vi "DataFinder_DisplaySignal_nointerps.vi"(8 "error in":errorcluster {"code" min=0 max=0}, 10 "result references":refnum<k20>[](array[refnum])) -> ()   [LabVIEW 2014]
doc: "Displays resulting signals as waveforms."
uses:
  <vilib>/DataFinder/DataTypes/property.ctl
  <vilib>/DataFinder/DataTypes/object type.ctl
  <vilib>/DataFinder/DataTypes/data type.ctl
  <vilib>/DataFinder/Get Property Values (Numeric Property).vi
  <vilib>/DataFinder/Get Property Values (Date Property).vi
  <vilib>/Utility/error.llb/DialogType.ctl
  <vilib>/DataFinder/NI_DataFinder Toolkit.lvlib
  <vilib>/DataFinder/Results to Waveforms (ddt).vi
  <vilib>/Analysis/NI_AALPro.lvlib
panel:
  out "Array":i32[](array[numeric])
  out "slope":dbl
  out "XY Graph 2":T1(graph)
  out "date/time string":string
  out "error out":errorcluster
  out "Timestamp":timestamp[](array[timestamp])
  out "property values":dbl[](array[numeric])
  out "XY Graph":T2(graph)
  out "Resulting Signals":dynamicdata(graph)
  out "error text":string=" INSTRUCTIONS:\r\rNormal Use:  When using subVIs that incorporate the error in/error out (or error I/O) structure, place this handler where you want to inform the user of an error, typically at the end of the I/O data path, as the last action of the program.  If the error in error? is ERROR, the handler creates a message describing the error and its source.  If the type of dialog = 1 (default), the message is displayed to the user, who can only acknowedge it.  If the type = 2, the user can acknowledge the message or abort execution; aborting a program with active I/O is not recommended.  If the type = 0, no message is displayed; this is used to process the error programmatically, and the error out cluster elements are wired to individual terminals for that reason.  \r\rOther Use:\n\r\nlocal testing.  To test the error code of a subVI or function that does not have the error I/O structure, you can wire its error code and a source string to the local error code and error source inputs.  If error in error? indicates no error and error code is not equal to 0, the local code and source are substituted for the error in values, and error? is set TRUE (ERROR)."
  in  "Close":bool
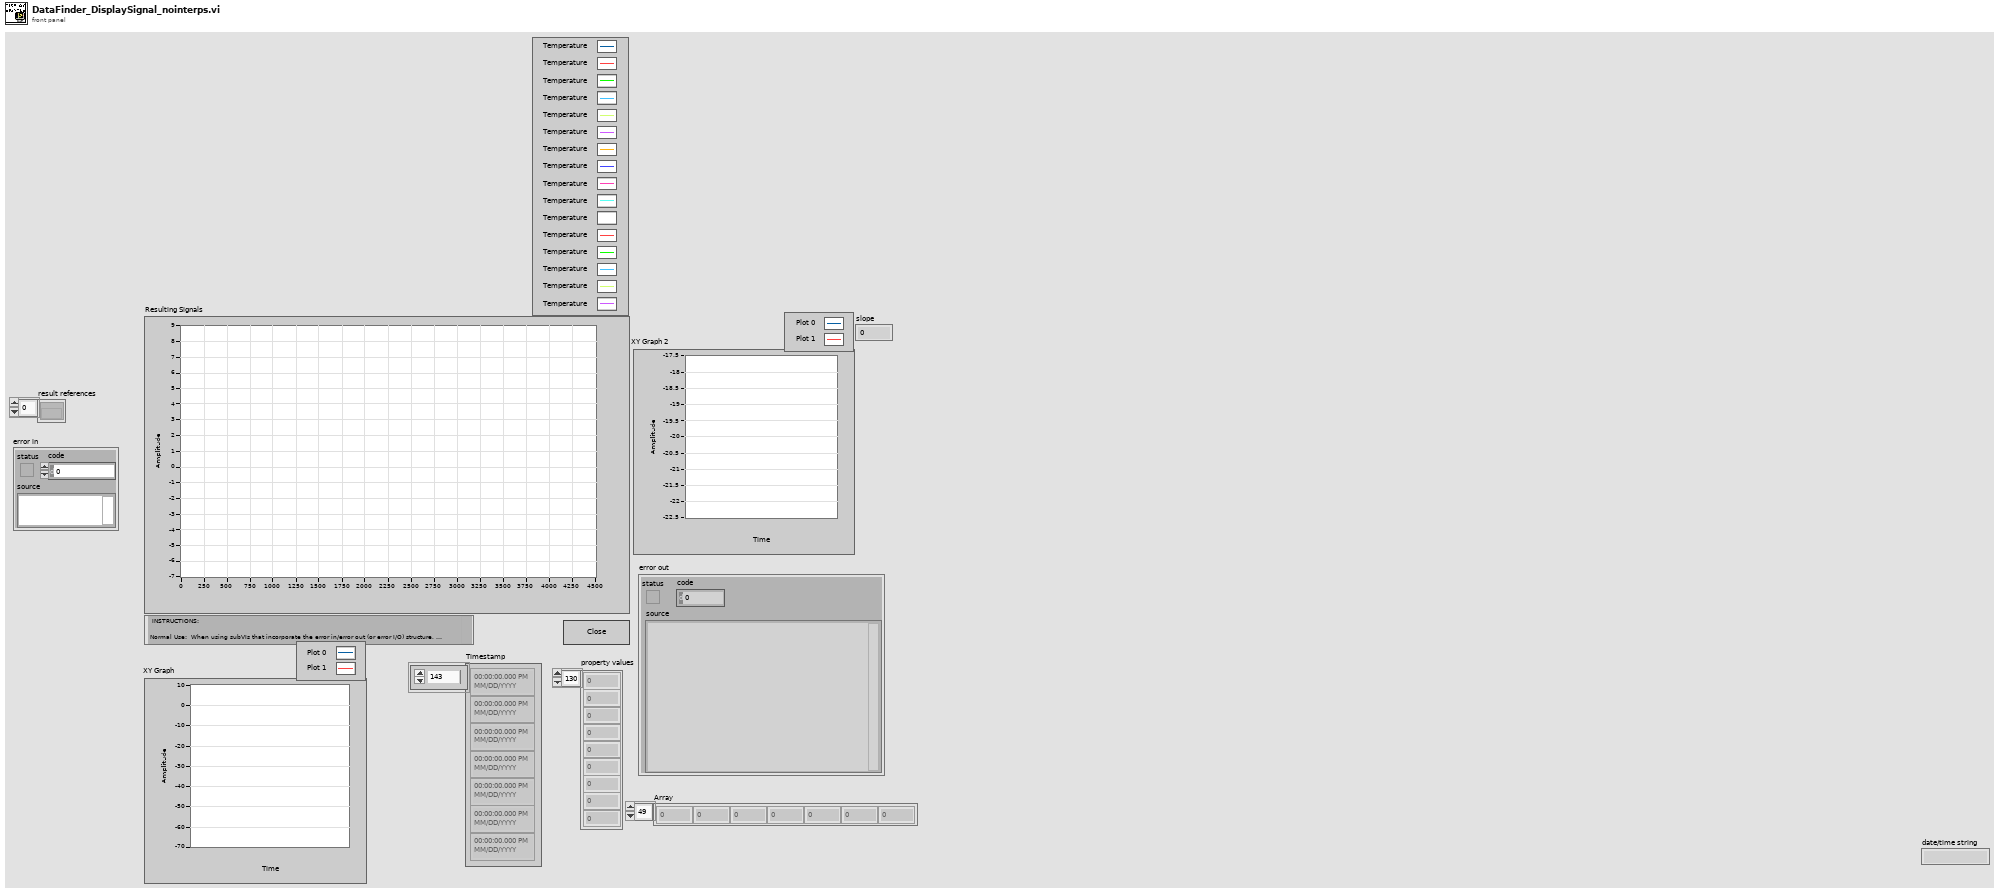
[diagram p1: front panel]
types:
  T1 = cluster{"property values":timestamp[], "Best Linear Fit":dbl[]}
  T2 = cluster{"property values":timestamp[], "Best Linear Fit":dbl[]}[]
  T3 = typedef "NI_DataFinder Toolkit.lvlib/property.ctl" = cluster{"object type":T4, "property name":string, "data type":T5}
  T4 = typedef "NI_DataFinder Toolkit.lvlib/object type.ctl" = u16
  T5 = typedef "NI_DataFinder Toolkit.lvlib/data type.ctl" = u16
  T6 = typedef "DialogType.ctl" = u16
  T7 = typedef "NI_DataFinder Controls.lvlib/DFSearchResult.ctl" = refnum<k20>
  T8 = cluster{"property values":timestamp[], "property values":dbl[]}
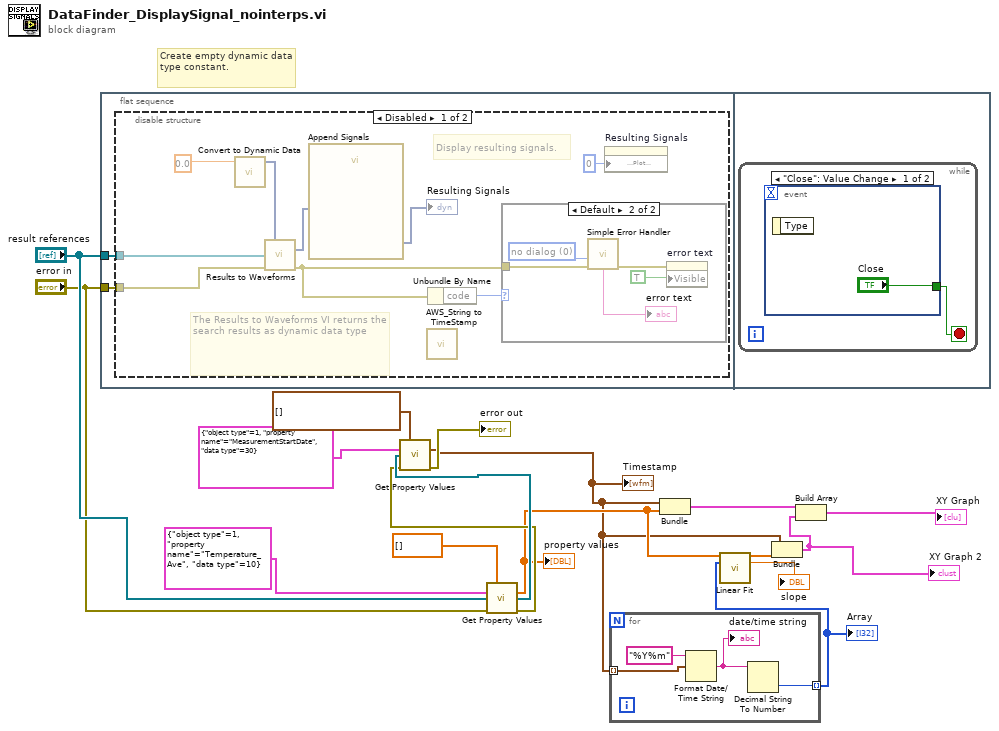
[diagram p0: block diagram]
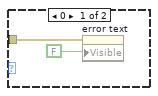
[diagram p2: hidden frame]
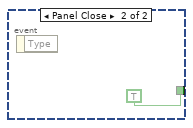
[diagram p4: hidden frame]
diagram:
  # "Create empty dynamic data type constant."
  n1 = flat-sequence {
    tunnel: "result references" -> [w19]
    tunnel: "error in" -> [w18]
    frame #0 {
      n2 = disable-structure shown="Disabled" {
        disable-tunnel: w19 -> [w26 _]
        disable-tunnel: w18 -> [w25 _]
        frame Disabled {
          # "The Results to Waveforms VI returns the search results as dynamic data type"
          # "Display resulting signals."
          n3 = call "Convert to Dynamic Data"("Double"=0.0) -> ("Dynamic Data Type"=w23:dynamicdata)  [unwired: 3 in]
          n4 = call-poly <vilib>:"Results to Waveforms.vi"("data type"=w23, "result references"=w26, "error in (no error)"=w25) -> ("signals out"=w22:dynamicdata, "error out"=w28:errorcluster)  [unwired: 11 out]
          n5 = call "Append Signals"("Input Signal A"=w22) -> ("Appended Signals"=→"Resulting Signals":dynamicdata)  [unwired: 9 in, 1 out]
          n6 = call "AWS_String to TimeStamp.vi"() -> ()  [unwired: 10 in, 1 out]
          n7 = Unbundle By Name(w28) -> ("code"=w27:i32)
          n8 = case shown="Default" w27 {
            tunnel: w28 -> [w29 w31]
            frame 0 {
              n9 = property on="error text" class="Str"(error in=w29, "Visible"=FALSE) -> ()  [unwired: 1 in, 2 out]
            }
            frame Default {
              w35 = T6 0 items=["no dialog", "OK message", "continue or stop message", "OK message + warnings", "continue/stop + warnings"] ("type of dialog (OK msg:1)")
              n10 = call <vilib>:"Simple Error Handler.vi"("type of dialog (OK msg:1)"=w35, "error in (no error)"=w31) -> ("error out"=w32:errorcluster, "message"=→"error text":string)  [unwired: 2 in, 4 out]
              n11 = property on="error text" class="Str"(error in=w32, "Visible"=TRUE) -> ()  [unwired: 1 in, 2 out]
            }
          }
          n12 = property on="Resulting Signals" class="WFGraph (strict)"("Plot.Plot Interpolation"=u8 0) -> ()  [unwired: 2 in, 2 out]
        }
        frame Enabled {
        }
      }
    }
    frame #1 {
      n13 = while {
        stop <- w36 stop-if-true
        n14 = event shown="[0] \"Close\": Value Change" {
          selector: _ -> [_ _]
          dyn-events: _ -> [_ _]
          timeout: _ -> [_ _]
          tunnel: ["Close" TRUE ("Cancel")] -> w36
          event "Close": Value Change {
            n15 = event-data() -> ()  [unwired: 1 in, 1 out]
          }
          event Panel Close {
            n16 = event-data() -> ()  [unwired: 1 in, 1 out]
          }
        }
      }
    }
  }
  n17 = call-poly <vilib>:"Get Property Values.vi"("data type"=dbl[] [], "property"=T3 {"object type"=1, "property name"="Temperature_Ave", "data type"=10}, "result references"="result references", "error in (no error)"="error in") -> ("property values"=w8:dbl[], "result references out"=w11:T7[], "error out"=w10:errorcluster)  [unwired: 9 in]
  "property values" <- w8
  n18 = call-poly <vilib>:"Get Property Values.vi"("data type"=timestamp[] [] ("Timestamp"), "property"=T3 {"object type"=1, "property name"="MeasurementStartDate", "data type"=30}, "result references"=w11, "error in (no error)"=w10) -> ("property values"=w4:timestamp[], "error out"=→"error out":errorcluster)  [unwired: 9 in, 1 out]
  "Timestamp" <- w4
  n19 = for {
    tunnel: [w40] -> w6 mode=indexing
    tunnel: w4 -> [w39] mode=indexing
    n20 = Format Date/Time String(time format string (%c)="%Y%m", seconds (now)=w39) -> (date/time string=w41:string)  [unwired: 1 in]
    "date/time string" <- w41
    n21 = Decimal String To Number(string=w41) -> (number=w40:i32)  [unwired: 2 in, 1 out]
  }
  "Array" <- w6
  n22 = Bundle("property values"=w4, "property values"=w8) -> (w5:T8)  [unwired: 1 in]
  n23 = call <vilib>:"Linear Fit.vi"("Y"=w8, "X"=w6) -> ("Best Linear Fit"=w7:dbl[], "slope"=→"slope":dbl)  [unwired: 9 in, 3 out]
  n24 = Bundle("property values"=w4, "Best Linear Fit"=w7) -> (w2:T1)  [unwired: 1 in]
  "XY Graph 2" <- w2
  n25 = Build Array(w5, w2) -> (→"XY Graph":T2)
